vi "calc_phasemap_from_stored_images_joe.vi"() -> ()   [LabVIEW 2011]
uses:
  <userlib>/_OpenG.lib/file/file.llb/Build Path - Traditional__ogtk.vi
  global_vars.vi
panel:
  in  "normalize":bool
  out "Phase Line (unwrapped)":dbl[](graph)
  out "unwrapped phase map":T1(plugin-control)
  out "u8_ar_phase map":u8[][](array[numeric])
  out "Phase Line (wrapped)":u8[](graph)
  in  "pick row for\nphase line plot":i32(slide) min=0 scale=0.0..499.0
  in  "calculate \nphase map":bool
  out "img_phase map":T1(plugin-control)
  out "current image":T1(plugin-control)
  out "Image Pixels":u8[][][](array[numeric])
  in  "current image":string="fringe"
  in  "pick input image":i32
  in  "phase map file name":string="orig.png"
  in  "EXP Folder Path":path=path "X:/Cloud Drives/Dropbox/Europhotonics/FringeMan/Image Storage/01_09/playing around" caption="Enter or select file path"
  in  "save phasemap":bool
  in  "read files":bool
  in  "Stop Button":bool
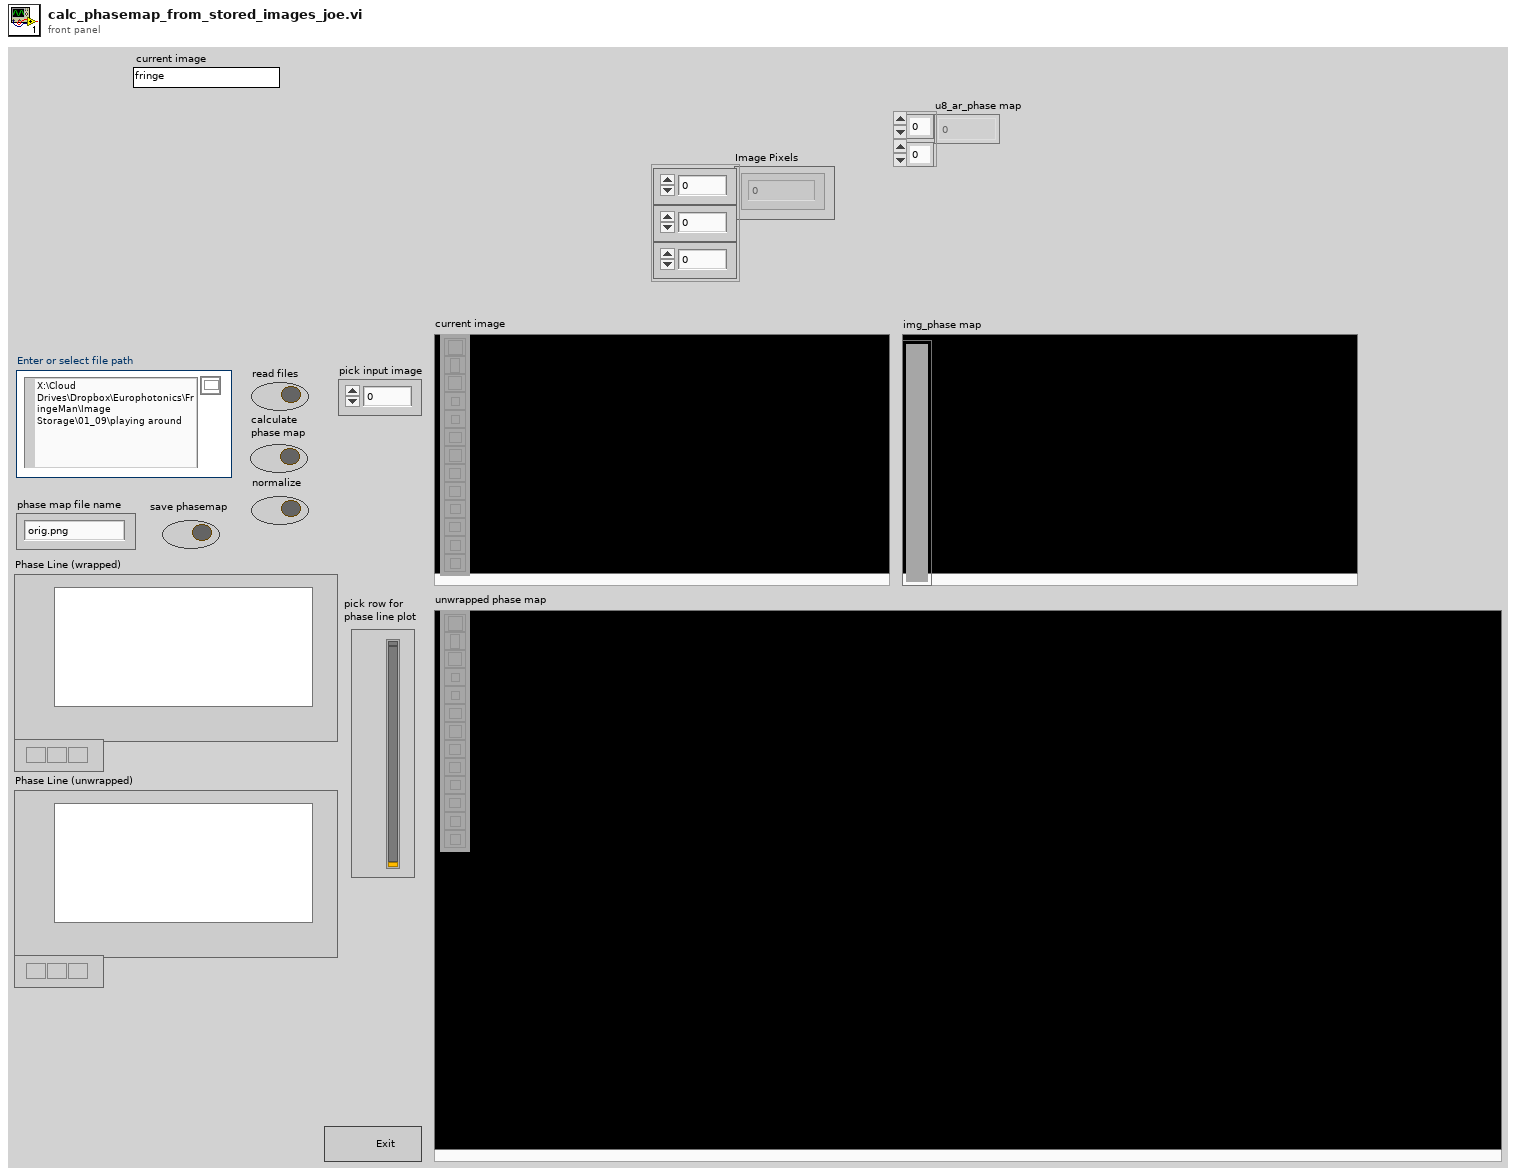
[diagram p1: front panel]
types:
  T1 = typedef "IMAQ Image.ctl" = refnum<image>
  T2 = typedef "Image Type" = u32
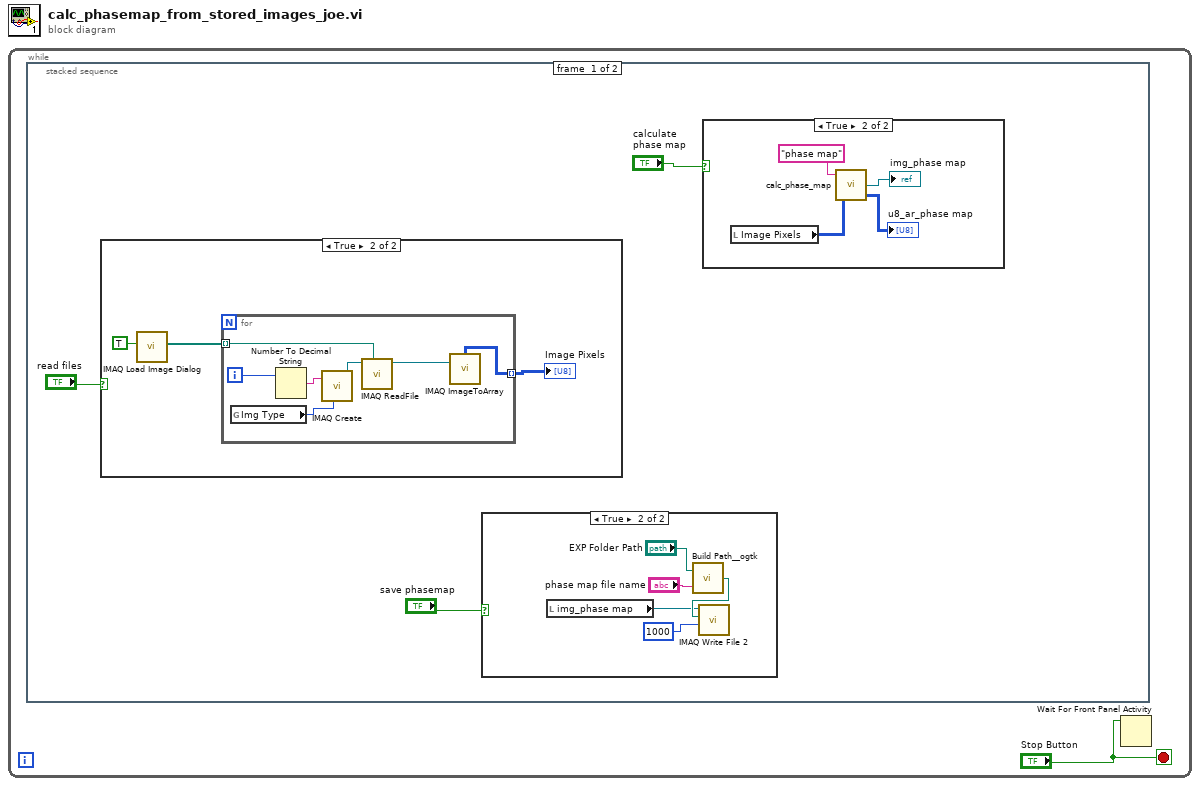
[diagram p0: block diagram]
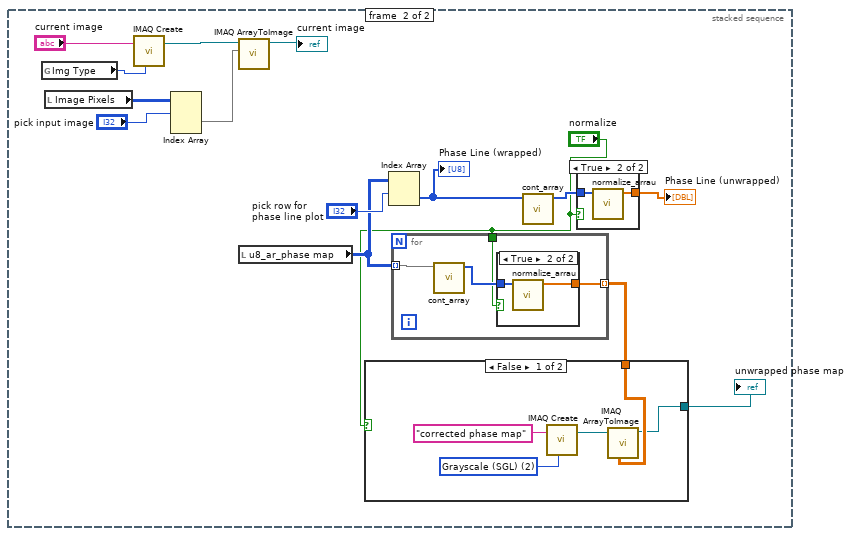
[diagram p5: hidden frame]
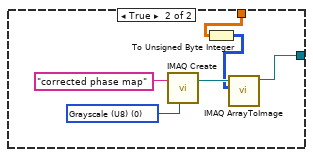
[diagram p6: hidden frame]
diagram:
  n1 = while {
    stop <- "Stop Button" stop-if-true
    n2 = stacked-sequence {
      frame #0 {
        n3 = case shown="True" "read files" {
          frame False {
          }
          frame True {
            n4 = call "IMAQ Load Image Dialog"("Multiple Files? (No)"=TRUE) -> ("Paths"=w16:path[])  [unwired: 8 in, 2 out]
            n5 = for {
              tunnel: w16 -> [w23] mode=indexing
              tunnel: [w18] -> w14 mode=indexing
              i -> [w22]
              n6 = global read "global_vars.vi" "Img Type"() -> (w17:T2)
              n7 = Number To Decimal String(number=w22) -> (decimal integer string=w21:string)  [unwired: 1 in]
              n8 = call "IMAQ Create"("Image Name"=w21, "Image Type"=w17) -> ("New Image"=w20:T1)  [unwired: 2 in, 2 out]
              n9 = call "IMAQ ReadFile"("File Path"=w23, "Image"=w20) -> ("Image Out"=w19:T1)  [unwired: 5 in, 4 out]
              n10 = call "IMAQ ImageToArray"("Image"=w19) -> ("Image Pixels (U8)"=w18:u8[][])  [unwired: 3 in, 4 out]
            }
            "Image Pixels" <- w14
          }
        }
        n11 = case shown="True" "save phasemap" {
          frame False {
          }
          frame True {
            n12 = local read "img_phase map"() -> (w9:T1)
            n13 = call-poly <userlib>:"Build Path__ogtk.vi"("name or relative path"="phase map file name", "base path"="EXP Folder Path") -> ("appended path"=w11:path)
            n14 = call-poly "IMAQ Write File 2"("Image Quality"=u32 1000, "File Path"=w11, "Image"=w9) -> ()  [unwired: 7 in, 2 out]
          }
        }
        n15 = case shown="True" "calculate \nphase map" {
          frame False {
          }
          frame True {
            n16 = local read "Image Pixels"() -> (w7:u8[][][])
            n17 = call "calc_phase_map.vi"("u8_ar_image_pixel_array"=w7, "image name"="phase map" ("String")) -> ("raw phase map array"=→"u8_ar_phase map":u8[][], "phase map"=→"img_phase map":T1)  [unwired: 2 in]
          }
        }
      }
      frame #1 {
        n18 = global read "global_vars.vi" "Img Type"() -> (w35:T2)
        n19 = local read "Image Pixels"() -> (w38:u8[][][])
        n20 = call "IMAQ Create"("Image Name"="current image", "Image Type"=w35) -> ("New Image"=w37:T1)  [unwired: 2 in, 2 out]
        n21 = Index Array(array=w38, index (dim 0)="pick input image") -> (element=w32:u8[][])  [unwired: 2 in]
        n22 = call "IMAQ ArrayToImage"("Image Pixels (U8)"=w32, "Image"=w37) -> ("Image Out"=→"current image":T1)  [unwired: 8 in, 1 out]
        n23 = local read "u8_ar_phase map"() -> (w29:u8[][])
        n24 = Index Array(array=w29, index (row)="pick row for\nphase line plot") -> (element=w30:u8[])  [unwired: 1 in]
        "Phase Line (wrapped)" <- w30
        n25 = for {
          tunnel: w29 -> [w56] mode=indexing
          tunnel: [w54] -> w25 mode=indexing
          tunnel: "normalize" -> [w53]
          n26 = call "cont_array.vi"("u8_ar_phase map"=w56) -> ("Array"=w55:i16[])  [unwired: 10 in]
          n27 = case shown="True" w53 {
            tunnel: w55 -> [w57 w59]
            tunnel: [w57 w58] -> w54
            frame False {
            }
            frame True {
              n28 = call "normalize_arrau.vi"("Array in"=w59) -> ("Array out"=w58:dbl[])  [unwired: 10 in]
            }
          }
        }
        n29 = case shown="False" "normalize" {
          tunnel: [w39 w49] -> w28
          tunnel: w25 -> [w40 w45]
          frame False {
            w42 = T2 2 items=["Grayscale (U8)", "Grayscale (I16)", "Grayscale (SGL)", "Complex (CSG)", "RGB (U32)", "HSL (U32)", "RGB (U64)", "Grayscale (U16)"] ("Image Type")
            n30 = call "IMAQ Create"("Image Name"="corrected phase map" ("corrected phase map"), "Image Type"=w42) -> ("New Image"=w43:T1)  [unwired: 2 in, 2 out]
            n31 = call "IMAQ ArrayToImage"("Image Pixels (Float)"=w40, "Image"=w43) -> ("Image Out"=w39:T1)  [unwired: 8 in, 1 out]
          }
          frame True {
            w47 = T2 0 items=["Grayscale (U8)", "Grayscale (I16)", "Grayscale (SGL)", "Complex (CSG)", "RGB (U32)", "HSL (U32)", "RGB (U64)", "Grayscale (U16)"] ("Image Type")
            n32 = call "IMAQ Create"("Image Name"="corrected phase map" ("corrected phase map"), "Image Type"=w47) -> ("New Image"=w48:T1)  [unwired: 2 in, 2 out]
            n33 = To Unsigned Byte Integer(number=w45) -> (unsigned 8bit integer=w44:u8[][])
            n34 = call "IMAQ ArrayToImage"("Image Pixels (U8)"=w44, "Image"=w48) -> ("Image Out"=w49:T1)  [unwired: 8 in, 1 out]
          }
        }
        "unwrapped phase map" <- w28
        n35 = call "cont_array.vi"("u8_ar_phase map"=w30) -> ("Array"=w27:i16[])  [unwired: 10 in]
        n36 = case shown="True" "normalize" {
          tunnel: w27 -> [w50 w52]
          tunnel: [w50 w51] -> w26
          frame False {
          }
          frame True {
            n37 = call "normalize_arrau.vi"("Array in"=w52) -> ("Array out"=w51:dbl[])  [unwired: 10 in]
          }
        }
        "Phase Line (unwrapped)" <- w26
      }
    }
    n38 = Wait For Front Panel Activity(3:"Stop Button") -> ()  [unwired: 2 in, 1 out]
  }
